vi "mxwScript_API_XMLRunAddOn.vi"(8 "error in (no error)":errorcluster, 9 "control values":T1[](array[typedef]), 10 "context":T2, 11 "VI path":path) -> (0 "error out":errorcluster, 3 "connection":T3)   [LabVIEW 2020]
doc: "Create encoded control name for connecting to a terminal on a generic node instead of to a control terminal. Terminal is specified by name. If multiple terminals with the same name exist, the first one is used.\n\nThis encoding works for both connected to and connected from terminals."
uses:
  codeGenAPISupport.llb/cgAPI_mxwScript_TemplateInfo.ctl
  codeGenAPISupport.llb/cgAPI_mxwScript_Wire_InputWireConnection.ctl
  codeGenAPISupport.llb/cgAPI_mxwScript_Parameter.ctl
  codeGenAPISupport.llb/cgAPI_mxwScript_RunContext.ctl
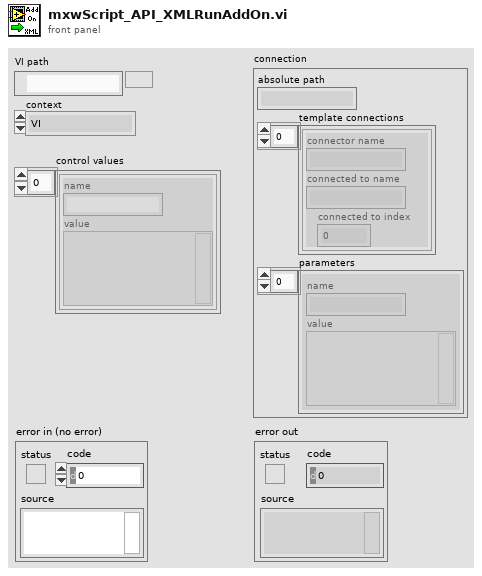
[diagram p1: front panel]
types:
  T1 = typedef "cgAPI_mxwScript_Parameter.ctl" = cluster{"name":string, "value":variant}
  T2 = typedef "cgAPI_mxwScript_RunContext.ctl" = enum16{"VI", "Engine"}
  T3 = typedef "cgAPI_mxwScript_TemplateInfo.ctl" = cluster{"absolute path":string, "template connections":T4[], "parameters":T1[]}
  T4 = typedef "cgAPI_mxwScript_Wire_InputWireConnection.ctl" = cluster{"connector name":string, "connected to name":string, "connected to index":i32}
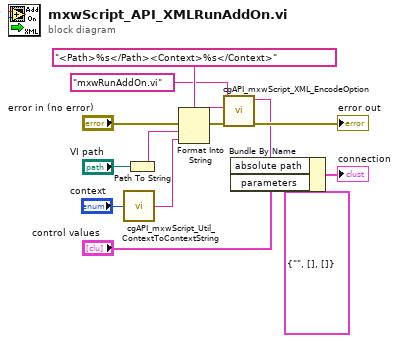
[diagram p0: block diagram]
diagram:
  n1 = call "cgAPI_mxwScript_Util_ContextToContextString.vi"("context"="context") -> ("contextString"=w7:string)  [unwired: 4 out]
  n2 = Path To String(path="VI path") -> (string=w6:string)
  n3 = Format Into String(format string="<Path>%s</Path><Context>%s</Context>" ("control name"), error in="error in (no error)", w6, w7) -> (resulting string=w11:string, error out=w12:errorcluster)  [unwired: 1 in]
  n4 = call "cgAPI_mxwScript_XML_EncodeOption.vi"("error in (no error)"=w12, "otherXML"=w11, "normalTextString"="mxwRunAddOn.vi") -> ("error out"=→"error out":errorcluster, "encodedString"=w3:string)  [unwired: 7 out]
  n5 = Bundle By Name(cluster=T3 {"absolute path"="", "template connections"=[], "parameters"=[]} ("connection"), "absolute path"=w3, "parameters"="control values") -> (→"connection":T3)
